vi "fgv.vi"(2 "error in (no error)":errorcluster, 3 "initial position":dbl, 4 "Enum":enum16{"init", "process 1", "process 2", "read"}(ring)) -> (0 "error out":errorcluster, 1 "new position":dbl)   [LabVIEW 2013]
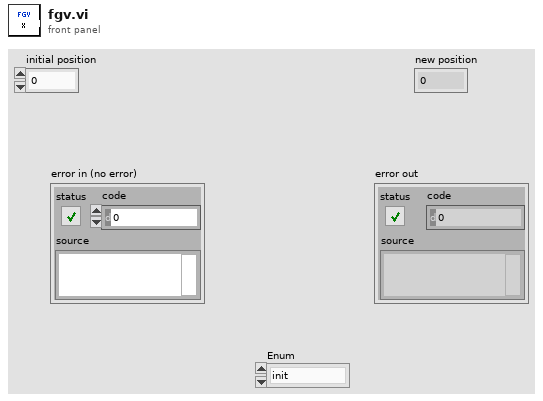
[diagram p1: front panel]
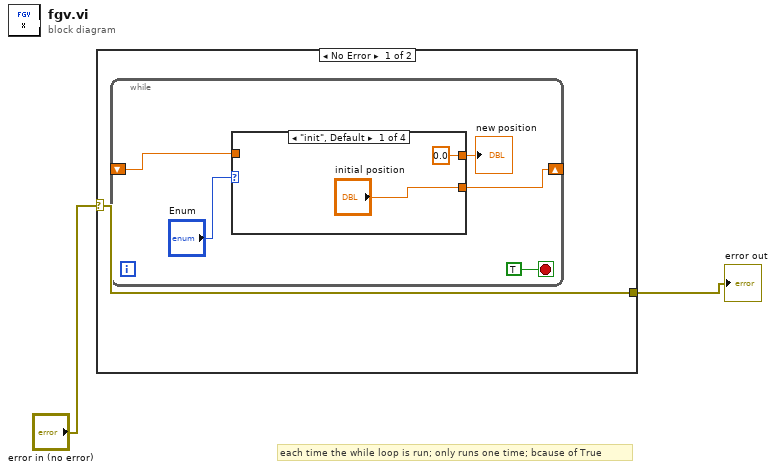
[diagram p0: block diagram]
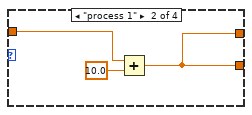
[diagram p2: hidden frame]
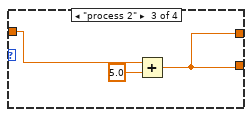
[diagram p3: hidden frame]
diagram:
  # "each time the while loop is run; only runs one time; bcause of True"
  n1 = case shown="No Error" "error in (no error)" {
    selector: "error in (no error)" -> [w3 w18]
    tunnel: [w3 w18] -> w1
    frame No Error {
      n2 = while {
        shift-right: [w6] -> _
        shift-left: _ -> [w5]
        stop <- TRUE stop-if-true
        n3 = case shown="\"init\", Default" "Enum" {
          tunnel: ["initial position" w11 w14 w17] -> w6
          tunnel: w5 -> [_ w12 w16 w17]
          tunnel: [0.0 w11 w14 w17] -> w4
          frame "init", Default {
          }
          frame "process 1" {
            n4 = Add(x=w12, y=10.0) -> (x+y=w11:dbl)
          }
          frame "process 2" {
            n5 = Add(x=w16, y=5.0) -> (x+y=w14:dbl)
          }
          frame "read" {
          }
        }
        "new position" <- w4
      }
    }
    frame Error {
    }
  }
  "error out" <- w1
